vi "PH_BeamlineController.PC _PA-Backreflection.vi"(0 "i ref in":refnum<vi>, 5 "error IO":errorcluster) -> (14 "i ref out":refnum<vi>, 19 "error out":errorcluster)   [LabVIEW 2014, in "PH_BeamlineController.lvlib"]
doc: "This VI sets incoming values to the GUI element."
uses:
  PH_BeamlineController.lvlib
  PH_Common/PH_Common.lvlib
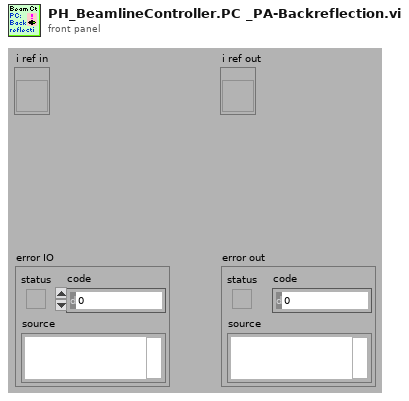
[diagram p1: front panel]
types:
  T1 = typedef "PH_StatusHandler.lvlib/PH_StatusHandler.Status.ctl" = i16
  T2 = typedef "PH_BeamlineController.lvlib/PH_BeamlineController.i attribute.ctl" = cluster{"Vacuum Exp LB":cluster{"Channel":string, "Limit [mbar]":dbl, "Pressure [mbar]":dbl, "GUI Ref":refnum<vi>}, "Sources":T3[], "PA DP Targets":T5[], "Path":cluster{"Source":T4, "PA DP Target":T6, "Target":T7}, "Targets":cluster{"Name":T7, "GUI Ref":refnum<vi>, "Current State":bool, "Wanted State":bool, "Enabled":bool}[], "Status Tags":cluster{"Name":string, "Status":T1}[], "special GUI Refs":T8}
  T3 = typedef "PH_BeamlineController.lvlib/PH_BeamlineController.Source Attributes.ctl" = cluster{"Name":T4, "GUI Ref":refnum<vi>, "Current State":bool, "Wanted State":bool}
  T4 = typedef "PH_BeamlineController.lvlib/PH_BeamlineController.Sources.ctl" = enum16{"None", "YLF", "fs-Frontend", "ns-Frontend", "YLF and ns-Frontend", "fs- and ns-Frontend"}
  T5 = typedef "PH_BeamlineController.lvlib/PH_BeamlineController.PA DP Target Attributes.ctl" = cluster{"Name":T6, "GUI Ref":refnum<vi>, "Current State":bool, "Wanted State":bool, "Enabled":bool}
  T6 = typedef "PH_BeamlineController.lvlib/PH_BeamlineController.PA DP Targets.ctl" = enum16{"None", "Dump PA Delayed Beam", "Dump PA Undelayed Beam", "Dumps PA Delayed and Undelayed Beam"}
  T7 = typedef "PH_BeamlineController.lvlib/PH_BeamlineController.Targets.ctl" = enum16{"None", "PreAmp", "Dump Exp Laserlab", "Exp Laserlab", "Calorimeter", "Dump Exp Laserbay", "Exp Laserbay", "Dump Exp Z6", "Exp Z6"}
  T8 = typedef "PH_BeamlineController.lvlib/PH_BeamlineController.special GUI Refs.ctl" = cluster{"PA-Backreflection-Meas":refnum<vi>, "fs_Synchrolock_Watch":refnum<vi>}
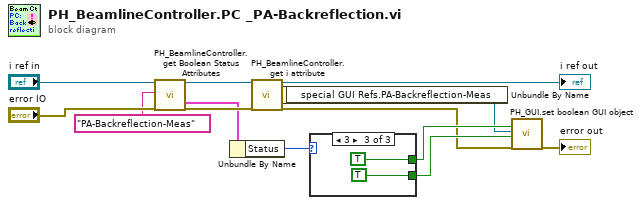
[diagram p0: block diagram]
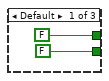
[diagram p2: hidden frame]
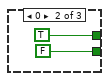
[diagram p3: hidden frame]
diagram:
  n1 = call "PH_BeamlineController.get Boolean Status Attributes.vi"("VI in"="i ref in", "Name"="PA-Backreflection-Meas" ("Instance PA Backreflection"), "error in (no error)"="error IO") -> ("VI out"=w4:refnum<vi>, "Tag"=w7:cluster{"Name":string, "Status":T1}, "error out"=w9:errorcluster)  [unwired: 11 in, 3 out]
  n2 = Unbundle By Name(w7) -> ("Status"=w6:T1)
  n3 = call "PH_BeamlineController.get i attribute.vi"("i ref in"=w4, "error in (no error)"=w9) -> ("i ref out"=→"i ref out":refnum<vi>, "i attribute"=w2:T2, "error out"=w5:errorcluster)  [unwired: 15 in]
  n4 = Unbundle By Name(w2) -> ("special GUI Refs.PA-Backreflection-Meas"=w1:refnum<vi>)
  n5 = case shown="3" w6 {
    tunnel: [FALSE TRUE TRUE] -> w11
    tunnel: [FALSE FALSE TRUE] -> w10
    frame Default {
    }
    frame 0 {
    }
    frame 3 {
    }
  }
  n6 = call "PH_GUI.set boolean GUI object.vi"("Visible (true)"=w11, "Boolean Knob GUI Ref"=w1, "Value"=w10, "error in (no error)"=w5) -> ("error out"=→"error out":errorcluster)  [unwired: 15 in]
